vi "Supported TC Types and Units.vi"() -> (2 "supported temperature units":cluster{"String":string, "Value":u16}[](array[cluster]), 3 "supported TC types":cluster{"String":string, "Value":u16}[](array[cluster]))   [LabVIEW 2019, in "Modules.lvlib" / "9210.lvclass"]
uses:
  9210.lvclass
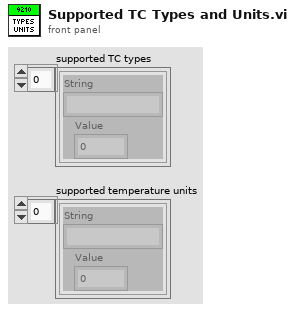
[diagram p1: front panel]
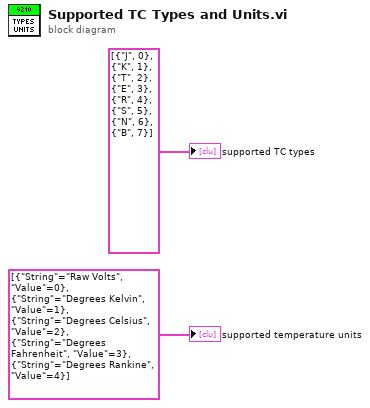
[diagram p0: block diagram]
diagram:
  "supported temperature units" <- cluster{"String":string, "Value":u16}[] [{"String"="Raw Volts", "Value"=0}, {"String"="Degrees Kelvin", "Value"=1}, {"String"="Degrees Celsius", "Value"=2}, {"String"="Degrees Fahrenheit", "Value"=3}, {"String"="Degrees Rankine", "Value"=4}] ("Units")
  "supported TC types" <- cluster{"String":string, "Value":u16}[] [{"String"="J", "Value"=0}, {"String"="K", "Value"=1}, {"String"="T", "Value"=2}, {"String"="E", "Value"=3}, {"String"="R", "Value"=4}, {"String"="S", "Value"=5}, {"String"="N", "Value"=6}, {"String"="B", "Value"=7}] ("Type")
